vi "sv_Convert to Even Angle Signal (Continuous Swept-Sine).vi"(0 "scaled signals [EU]":waveform(dbl)[](array[waveform]), 2 "reset? (F)":bool, 5 "new sample time [s]":dbl[](array[numeric]), 7 "new samples/rev":dbl, 11 "error in (no error)":errorcluster, 12 "stop band attenuation [dB]":dbl=96.0) -> (4 "even-angle signals":cluster{"r0":dbl, "dr":dbl, "Y":dbl[]}[](array[cluster]) {"r0" format="%.2p"; "dr" format="%.2p"; "Y" format="%.2f"}, 6 "even-angle channel info":T1[](array[typedef]) {"channel info"."pregain" format="%.2f"; "channel info"."weighting filter" items=["Linear", "A-weighting", "B-weighting", "C-weighting", "ITU-R 468-4", "Dolby", "CCITT", "C-message", "Wb", "Wc", "Wd", "We", "Wf", "Wh", "Wj", "Wk", "Wm", "AES17 20 kHz lowpass", "AES17 40 kHz lowpass", "AES17 20 kHz highpass", "AES17 40 kHz highpass"]; "channel info"."dB reference" format="%^.1e"; "channel info"."engineering units" items=["custom..."=0, "V"=1, "A"=21, "C"=30, "pC"=31, "s"=32, "-"=29, "Pa"=2, "N"=20, "g"=3, "m/s^2"=4, "m/s"=5, "m"=6, "mm/s"=12, "mm"=13, "micron/s"=14, "micron"=15, "in/s^2"=7, "in/s"=8, "in"=9, "mil/s"=10, "mil"=11, "rad/s^2"=16, "rad/s"=17, "rad"=18, "deg/s^2"=26, "deg/s"=27, "deg"=28, "RPM"=22, "cycle/s^2"=23, "Hz"=24, "cycle"=25, "strain"=19]; "channel info"."sensor sensitivity" format="%#_5f"}, 8 "even-angle position info":T5, 14 "actual max order":dbl, 15 "error out":errorcluster)   [LabVIEW 2017, in "SoundVib_ContSweptSine.lvlib"]
doc: "Converts an even-time-spaced scaled signal to an even-angle-spaced signal by resampling the acquired signal. The output signal is synchronous to the rotational speed with a constant number of samples per revolution. The data type you wire to the <B>scaled signal [EU]</B> input determines the polymorphic instance to use."
uses:
  <vilib>/addons/Sound and Vibration/svt_Continuous Swept Sine/SoundVib_ContSweptSine.lvlib
  <vilib>/addons/Sound and Vibration/Order Analysis/Misc/OAT Position Info.ctl
  <vilib>/addons/_NISVFA/_Shared subVIs/Controls/svc_Resampled Channel Info.ctl
  <vilib>/addons/_NISVFA/_Shared subVIs/Controls/svc_Channel Info.ctl
  <vilib>/addons/_NISVFA/_Shared subVIs/Controls/svc_Engineering Units Text Ring.ctl
  <vilib>/addons/_NISVFA/_Shared subVIs/Controls/svc_Weighting Filter Text Ring.ctl
  <vilib>/addons/_NISVFA/_Shared subVIs/Common/svc_Check for Waveform Parameter Continuity (no state).vi
  <vilib>/addons/_NISVFA/_Shared subVIs/Common/svc_Engineering Units to Unit Label.vi
  <vilib>/addons/_NISVFA/_Shared subVIs/Common/svc_Unit Label to Engineering Units.vi
  <vilib>/addons/Sound and Vibration/Order Analysis/Resample Order Tracking/SoundVib_Resampling.lvlib
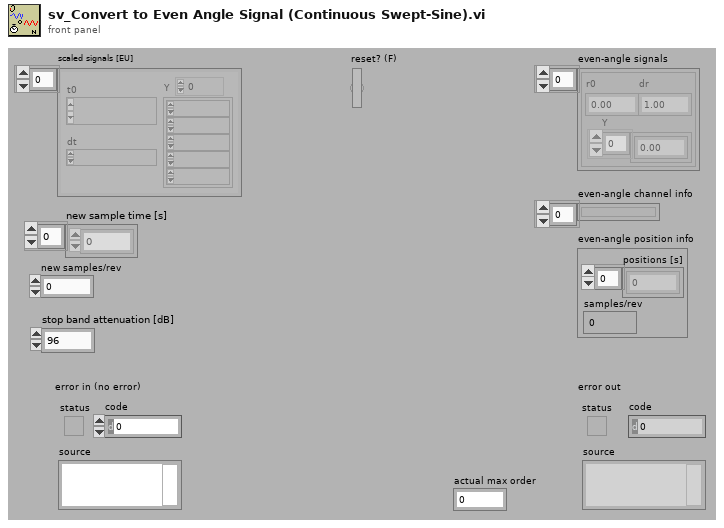
[diagram p1: front panel]
types:
  T1 = typedef "svc_Resampled Channel Info.ctl" = cluster{"channel name":string, "description":string, " channel info":T2}
  T2 = typedef "svc_Channel Info.ctl" = cluster{"sensor sensitivity":dbl, "engineering units":T3, "dB reference":dbl, "custom label":string, "weighting filter":T4, "pregain":dbl}
  T3 = typedef "svc_Engineering Units Text Ring.ctl" = u16
  T4 = typedef "svc_Weighting Filter Text Ring.ctl" = u16
  T5 = typedef "OAT Position Info.ctl" = cluster{"positions [s]":dbl[], "samples/rev":dbl}
  T6 = cluster{"dt equal":bool, "array length equal":bool, "number channels change":bool}
  T7 = cluster{"dt":bool, "t0 continuity":bool, "array length":bool, "channel info":bool, "name":bool}
  T8 = typedef "OAT Resample Filter Prototype.ctl" = cluster{"left wing":dbl[], "increment":dbl[], "max dec":i32, "timing jitter":enum32{"Interpolation", "Rounding"}, "band limiting?":bool}
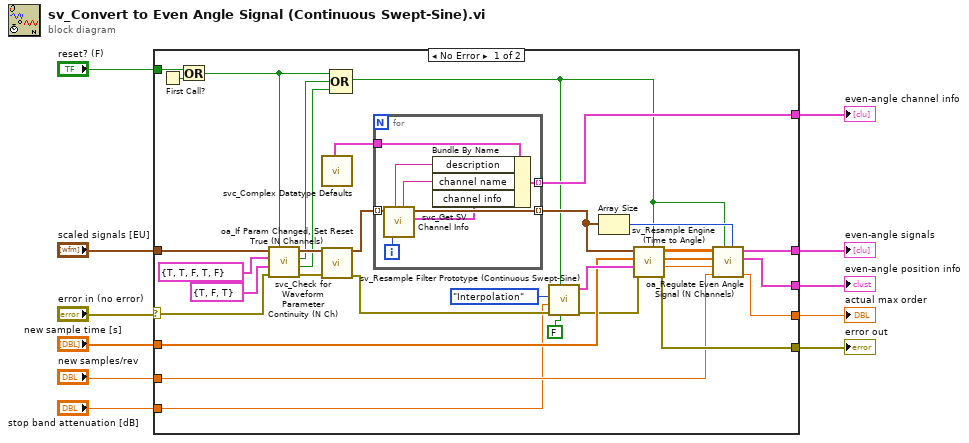
[diagram p0: block diagram]
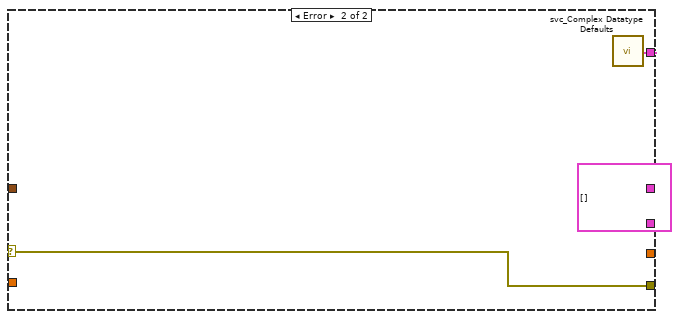
[diagram p2: hidden frame]
diagram:
  n1 = case shown="No Error" "error in (no error)" {
    selector: "error in (no error)" -> [w29 w55]
    tunnel: [w23 cluster{dbl, dbl, "Y":dbl[]}[] []] -> w10
    tunnel: [w42 w55] -> w11
    tunnel: [w35 w52] -> w9
    tunnel: [w22 _] -> w8
    tunnel: [w21 _] -> w7
    tunnel: "scaled signals [EU]" -> [w34 _]
    tunnel: "reset? (F)" -> [w37 _]
    tunnel: "new sample time [s]" -> [w19 _]
    tunnel: "new samples/rev" -> [w16 _]
    tunnel: "stop band attenuation [dB]" -> [w15 _]
    frame No Error {
      n2 = First Call?() -> (First Call?: T/F=w40:bool)
      n3 = Or(x=w37, y=w40) -> (x .or. y?=w32:bool)
      n4 = call <vilib>:"svc_Check for Waveform Parameter Continuity (N Ch).vi"("restart averaging (F)"=w32, "error in (no error)"=w29, "checks for multichannel parameters"=T6 {"dt equal"=TRUE, "array length equal"=FALSE, "number channels change"=TRUE}, "checks for channel parameter change"=T7 {"dt"=TRUE, "t0 continuity"=TRUE, "array length"=FALSE, "channel info"=TRUE, "name"=FALSE}, "scaled signal(s)"=w34) -> ("error out"=w28:errorcluster, "multichannel parameter changed"=w30:bool, "waveform parameter changed"=w31:bool, "dup scaled signal(s)"=w33:waveform(dbl)[])  [unwired: 3 out]
      n5 = call <vilib>:"svc_Complex Datatype Defaults.vi"() -> ("resampled channel info"=w12:T1)  [unwired: 11 in, 8 out]
      n6 = call <vilib>:"oa_If Param Changed, Set Reset True (N Channels).vi"("scaled signals in [EU]"=w33, "error in (no error)"=w28) -> ("scaled signals out [EU]"=w39:waveform(dbl)[], "error out"=w36:errorcluster)  [unwired: 7 in, 5 out]
      n7 = Compound Arithmetic op=OR(w32, w31, w30) -> (w18:bool)
      n8 = for {
        tunnel: w39 -> [w51] mode=indexing
        tunnel: [w50] -> w20 mode=indexing
        tunnel: [w49] -> w35 mode=indexing
        tunnel: w12 -> [w44]
        i -> [w46]
        n9 = call <vilib>:"svc_Get SV Channel Info.vi"("channel index"=w46, "scaled signal [EU]"=w51) -> ("channel info"=w48:T2, "dup scaled signal [EU]"=w50:waveform(dbl), "channel name"=w45:string, "channel description"=w47:string)  [unwired: 4 in, 2 out]
        n10 = Bundle By Name(cluster=w44, "description"=w47, "channel name"=w45, "channel info"=w48) -> (w49:T1)
      }
      n11 = call <vilib>:"sv_Resample Filter Prototype (Continuous Swept-Sine).vi"("alias free"=FALSE ("alias protect in final transition"), "reset? (True)"=w18, "error in (no error)"=w36, "stop band attenuation [dB]"=w15, "timing jitter"=enum32{"Interpolation", "Rounding"}."Interpolation") -> ("error out"=w17:errorcluster, "filter prototype"=w41:T8)  [unwired: 4 in, 1 out]
      n12 = Array Size(array=w20) -> (size(s)=w27:i32)
      n13 = call <vilib>:"sv_Resample Engine (Time to Angle).vi"("reset? (True)"=w18, "error in (no error)"=w17, "filter prototype"=w41, "time"=w19, "scaled signals (EU)"=w20) -> ("error out"=w42:errorcluster, "offset"=w24:dbl, "time stamps"=w25:dbl[], "Y"=w26:dbl[][])  [unwired: 3 in]
      n14 = call <vilib>:"oa_Regulate Even Angle Signal (N Channels).vi"("# of ch"=w27, "reset?"=w18, "samples/rev"=w16, "offset"=w24, "time stamps"=w25, "Data"=w26) -> ("actual max order"=w21:dbl, "even-angle position info"=w22:T5, "even-angle signals"=w23:cluster{"r0":dbl, "dr":dbl, "Y":dbl[]}[])  [unwired: 3 in]
    }
    frame Error {
      n15 = call <vilib>:"svc_Complex Datatype Defaults.vi"() -> ("resampled channel info"=w54:T1)  [unwired: 11 in, 8 out]
      n16 = Build Array(w54) -> (w52:T1[])
    }
  }
  "even-angle position info" <- w8
  "error out" <- w11
  "even-angle signals" <- w10
  "even-angle channel info" <- w9
  "actual max order" <- w7
